vi "FlatToRichProtocol_Response.vi"(5 "OutputClusterType":T1, 11 "InputCluster":T3) -> (3 "OutputCluster":T1)   [LabVIEW 2021, in "Unary_server.lvlib"]
uses:
  Unary_server.lvlib
  Protocol_Response_Flat.ctl
  Protocol_Request_Flat.ctl
  Protocol_Response.ctl
  Protocol_Request.ctl
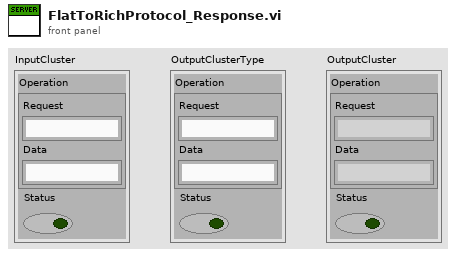
[diagram p1: front panel]
types:
  T1 = typedef "Unary_server.lvlib/Protocol_Response.ctl" = cluster{"Operation":T2, "Status":bool}
  T2 = typedef "Unary_server.lvlib/Protocol_Request.ctl" = cluster{"Request":string, "Data":string}
  T3 = typedef "Unary_server.lvlib/Protocol_Response_Flat.ctl" = cluster{"Operation":T4, "Status":bool}
  T4 = typedef "Unary_server.lvlib/Protocol_Request_Flat.ctl" = cluster{"Request":string, "Data":string}
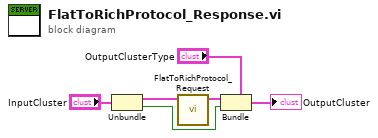
[diagram p0: block diagram]
diagram:
  n1 = Unbundle "Unbundle"("InputCluster") -> ("Operation"=w3:T4, "Status"=w1:bool)
  n2 = call "FlatToRichProtocol_Request.vi"("InputCluster"=w3) -> ("OutputCluster"=w2:T2)  [unwired: 10 in]
  n3 = Bundle "Bundle"(cluster="OutputClusterType", "Operation"=w2, "Status"=w1) -> (→"OutputCluster":T1)
